vi "Delete Icon Editor Source Files.vi"(8 "error in":errorcluster) -> (0 "error out":errorcluster)   [LabVIEW 2020]
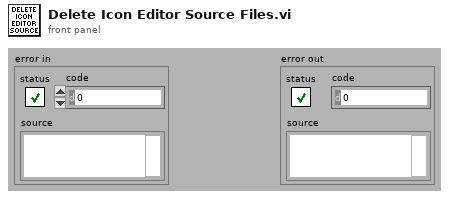
[diagram p1: front panel]
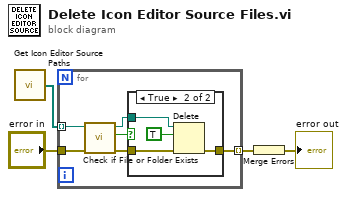
[diagram p0: block diagram]
diagram:
  n1 = call "Get Icon Editor Source Paths.vi"() -> ("IconEditorSourcePaths"=w3:path[])  [unwired: 1 in]
  n2 = for {
    tunnel: w3 -> [w9] mode=indexing
    tunnel: "error in" -> [w8]
    tunnel: [w10] -> w4 mode=indexing
    n3 = call <vilib>:"Check if File or Folder Exists.vi"("error in (no error)"=w8, "path"=w9) -> ("error out"=w7:errorcluster, "file or folder exists?"=w6:bool, "dup path"=w5:path)  [unwired: 7 in]
    n4 = case shown="True" w6 {
      tunnel: w7 -> [w11 w15]
      tunnel: [w11 w14] -> w10
      tunnel: w5 -> [_ w12]
      frame False {
      }
      frame True {
        n5 = Delete(path (use dialog)=w12, entire hierarchy (F)=TRUE, error in=w15) -> (error out=w14:errorcluster)  [unwired: 2 in, 2 out]
      }
    }
  }
  n6 = Merge Errors(w4) -> (→"error out":errorcluster)
